vi "Set_VI_Ref.vi"(8 "error in (no error)":errorcluster, 11 "Class 2 in":refnum<class "Class 2.lvclass">) -> (0 "error out":errorcluster, 2 "Core_Reference_VI out":refnum<vi>, 3 "Class 2 out":refnum<class "Class 2.lvclass">)   [LabVIEW 2021, in "Class 2.lvclass"]
uses:
  Class 2.lvclass
  Modules/Sample_Panel_2.vi
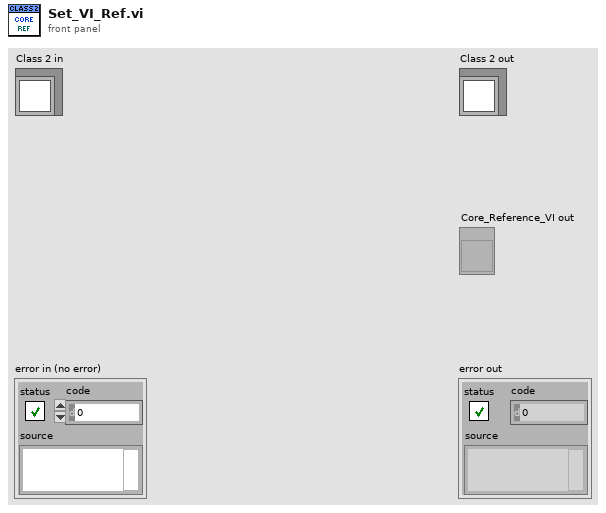
[diagram p1: front panel]
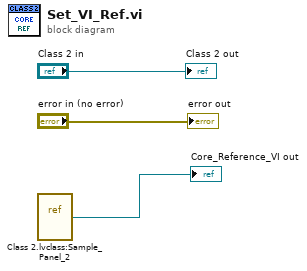
[diagram p0: block diagram]
diagram:
  n1 = vi-ref "Class 2.lvclass:Sample_Panel_2.vi"() -> (→"Core_Reference_VI out":refnum<vi>)
  "error out" <- "error in (no error)"
  "Class 2 out" <- "Class 2 in"
